vi "LoadXMLString__slk_msxml.vi"(0 "document in":refnum<class "msxml document.lvclass">, 1 "xml String":string, 11 "error in (no error)":errorcluster, 12 "validate on parse (F)":bool) -> (4 "document out":refnum<class "msxml document.lvclass">, 15 "error out":errorcluster)   [LabVIEW 2020, in "MSXML.lvlib" / "msxml document.lvclass"]
doc: "Loads an XML file to MSXML Document object and allows you to configure the XML parser to validate the file against a schema or DTD (Document Type Definition)."
uses:
  msxml document.lvclass
  msxml document.lvclass/msxml document.ctl
panel:
  # "LoadDocument__slk_msxml.vi\n\nLoads an XML file to MSXML Document object and allows you to configure the XML parser to validate the file against a schema or DTD (Document Type Definition).\n\nNOTICE -- YOU MUST LEAVE THIS NOTICE IN PLACE.\n\nCopyright (c) 2004-2010 Shawn Liu <shawn.liu.cn@gmail.com>\n\nAll rights reserved."
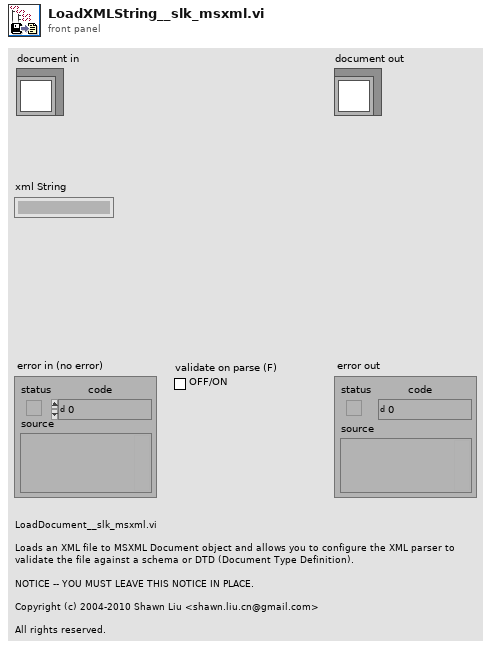
[diagram p1: front panel]
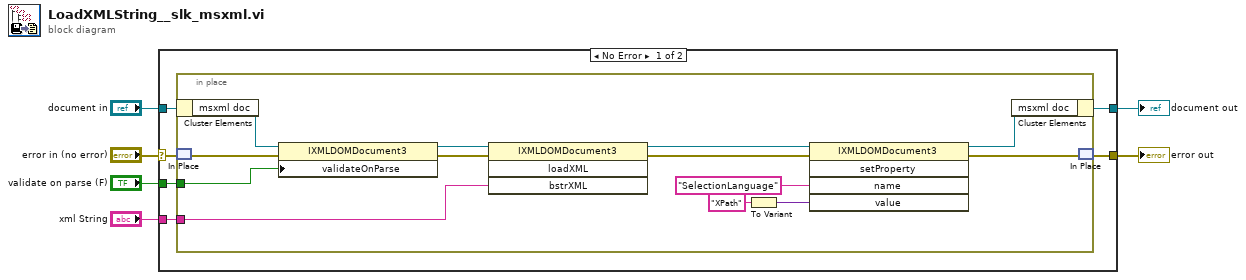
[diagram p0: block diagram]
diagram:
  n1 = case shown="No Error" "error in (no error)" {
    selector: "error in (no error)" -> [w9 w27]
    tunnel: [w8 w27] -> w3
    tunnel: [w7 w26] -> w5
    tunnel: "document in" -> [w10 w26]
    tunnel: "validate on parse (F)" -> [w12 _]
    tunnel: "xml String" -> [w11 _]
    frame No Error {
      n2 = in-place {
        in-place-border: w12 -> [w18]
        in-place-border: w11 -> [w13]
        n3 = in-place-cluster #1(w10) -> ("msxml doc"=w17:refnum<k7>)
        n4 = in-place-match #2(w9) -> (w15:errorcluster)
        n5 = property on="Property Node" class="IXMLDOMDocument3"(reference=w17, error in=w15, "validateOnParse"=w18) -> (reference out=w19:refnum<k7>, error out=w20:errorcluster)
        n6 = invoke on="Invoke Node" class="IXMLDOMDocument3" method="loadXML"(reference=w19, error in=w20, "bstrXML"=w13) -> (reference out=w25:refnum<k7>, error out=w24:errorcluster)  [unwired: 1 in, 2 out]
        n7 = To Variant(anything="XPath") -> (Variant=w21:variant)
        n8 = invoke on="Invoke Node" class="IXMLDOMDocument3" method="setProperty"(reference=w25, error in=w24, "name"="SelectionLanguage", "value"=w21) -> (reference out=w16:refnum<k7>, error out=w14:errorcluster)  [unwired: 1 in, 3 out]
        n9 = in-place-cluster #1("msxml doc"=w16) -> (w7:refnum<class "msxml document.lvclass">)
        n10 = in-place-match #2(w14) -> (w8:errorcluster)
      }
    }
    frame Error {
    }
  }
  "document out" <- w5
  "error out" <- w3
